vi "getInstrName.vi"(2 "ctlref":T1, 3 "abbr?":string) -> (0 "ctlref out":T1, 1 "name":string)   [LabVIEW 2017]
uses:
  RefArray/RefArray.ctl
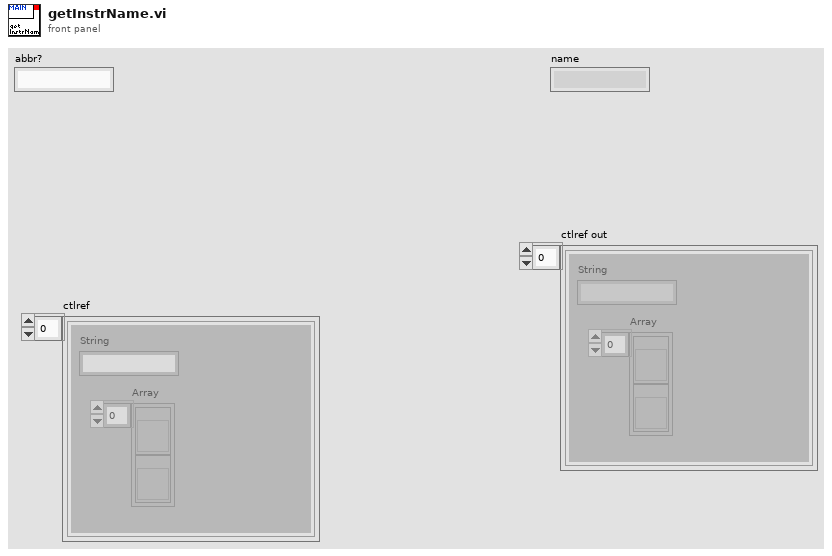
[diagram p1: front panel]
types:
  T1 = typedef "RefArray.ctl" = cluster{"String":string, "Array":refnum<vi>[]}[]
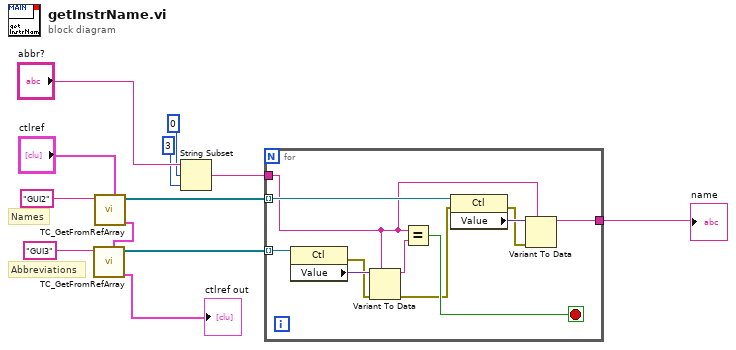
[diagram p0: block diagram]
diagram:
  # "Names"
  # "Abbreviations"
  n1 = call "TC_GetFromRefArray.vi"("arrayIn"="ctlref", "NameToFind"="GUI2") -> ("arrayOut"=w9:T1, "refArray"=w10:refnum<vi>[])  [unwired: 8 in]
  n2 = call "TC_GetFromRefArray.vi"("arrayIn"=w9, "NameToFind"="GUI3") -> ("arrayOut"=→"ctlref out":T1, "refArray"=w7:refnum<vi>[])  [unwired: 8 in]
  n3 = String Subset(string="abbr?", offset (0)=0, length (rest)=3) -> (substring=w3:string)
  n4 = for {
    tunnel: w10 -> [w19] mode=indexing
    tunnel: w7 -> [w23] mode=indexing
    tunnel: w3 -> [w14]
    tunnel: [w13] -> w2
    stop <- w20 stop-if-true
    n5 = property class="Ctl"(reference=w23) -> (error out=w15:errorcluster, "Value"=w22:variant)  [unwired: 1 in, 1 out]
    n6 = Variant To Data(error in=w15, type=w14, Variant=w22) -> (data=w21:string, error out=w16:errorcluster)
    n7 = Equal?(x=w14, y=w21) -> (x = y?=w20:bool)
    n8 = property class="Ctl"(reference=w19, error in=w16) -> (error out=w17:errorcluster, "Value"=w18:variant)  [unwired: 1 out]
    n9 = Variant To Data(error in=w17, type=w14, Variant=w18) -> (data=w13:string)  [unwired: 1 out]
  }
  "name" <- w2
